vi "Copy Member Data from Target.vi"(7 "AppInst":refnum<vi>, 8 "error in (no error)":errorcluster, 11 "Target Method path":path) -> (0 "error out":errorcluster, 1 "Wiring Rules":T1(array[ring]), 2 "Controls[]":refnum<vi>[](array[refnum]), 3 "Target Method Ref":refnum<vi>)   [LabVIEW 2020, in "Message Maker.lvlib"]
uses:
  Message Maker.lvlib
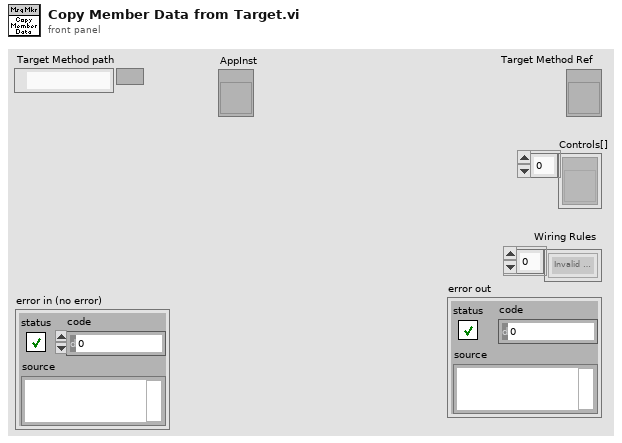
[diagram p1: front panel]
types:
  T1 = enum16{"Invalid Wire Rule", "Required", "Recommended", "Optional", "Dynamic Dispatch"}[]
  T2 = typedef "LVRectTypeDef.ctl" = cluster{"Left":i16, "Top":i16, "Right":i16, "Bottom":i16}
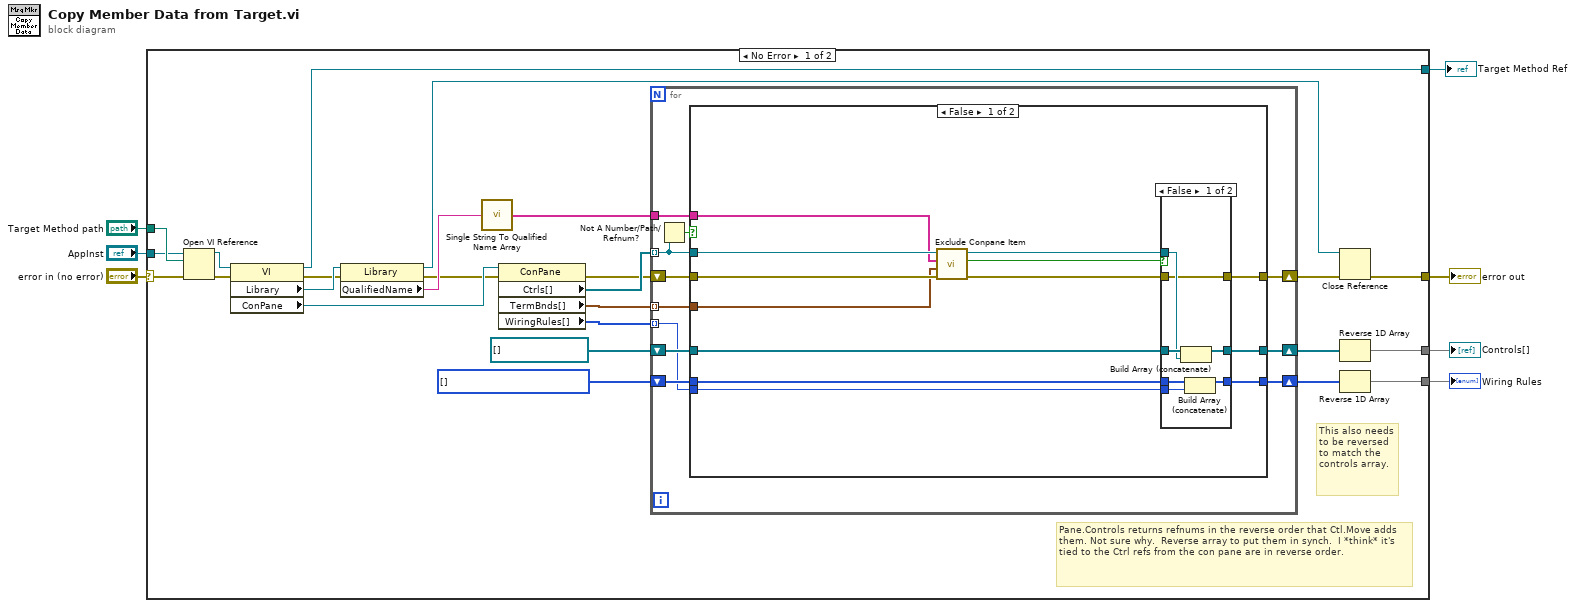
[diagram p0: block diagram]
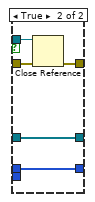
[diagram p2: hidden frame]
diagram:
  n1 = case shown="No Error" "error in (no error)" {
    selector: "error in (no error)" -> [w27 w72]
    tunnel: "Target Method path" -> [w28 _]
    tunnel: [w11 w72] -> w6
    tunnel: "AppInst" -> [w13 _]
    tunnel: [w8 _] -> w3
    tunnel: [w14 _] -> w2
    tunnel: [w12 _] -> w1
    frame No Error {
      w24 = T1 [] items=["Invalid Wire Rule", "Required", "Recommended", "Optional", "Dynamic Dispatch"] ("WiringRules[]")
      # "This also needs\nto be reversed to match the controls array."
      # "Pane.Controls returns refnums in the reverse order that Ctl.Move adds them. Not sure why.  Reverse array to put them in synch.  I *think* it's tied to the Ctrl refs from the con pane are in reverse order."
      n2 = Open VI Reference(application reference (local)=w13, vi path=w28, error in (no error)=w27) -> (vi reference=w29:refnum<vi>, error out=w30:errorcluster)  [unwired: 3 in]
      n3 = property class="VI"(reference=w29, error in=w30) -> (reference out=w12:refnum<vi>, error out=w31:errorcluster, "Library"=w32:refnum<vi>, "ConPane"=w22:refnum<vi>)
      n4 = property class="Library"(reference=w32, error in=w31) -> (reference out=w10:refnum<vi>, error out=w9:errorcluster, "QualifiedName"=w20:string)
      n5 = call <vilib>:"Single String To Qualified Name Array.vi"("Fully Qualified String"=w20) -> ("Fully Qualified Array"=w19:string[])
      n6 = property class="ConPane"(reference=w22, error in=w9) -> (error out=w18:errorcluster, "Ctrls[]"=w25:refnum<vi>[], "TermBnds[]"=w21:T2[], "WiringRules[]"=w23:T1)  [unwired: 1 out]
      n7 = for {
        tunnel: w25 -> [w38] mode=indexing
        tunnel: w19 -> [w43]
        shift-right: [w39] -> w17
        shift-left: w18 -> [w42]
        shift-right: [w40] -> w15
        shift-left: refnum<vi>[] [] ("Controls[]") -> [w41]
        shift-right: [w35] -> w16
        shift-left: w24 -> [w36]
        tunnel: w23 -> [w34] mode=indexing
        tunnel: w21 -> [w33] mode=indexing
        n8 = Not A Number/Path/Refnum?(number/path/refnum=w38) -> (NaN/Path/Refnum?=w37:bool)
        n9 = case shown="False" w37 {
          tunnel: w38 -> [w56 _]
          tunnel: w43 -> [w44 _]
          tunnel: w42 -> [w54 w71]
          tunnel: w41 -> [w52 w70]
          tunnel: [w51 w70] -> w40
          tunnel: [w50 w71] -> w39
          tunnel: w36 -> [w48 w69]
          tunnel: [w47 w69] -> w35
          tunnel: w34 -> [w46 _]
          tunnel: w33 -> [w45 _]
          frame False {
            n10 = call "Exclude Conpane Item.vi"("error in (no error)"=w54, "Rectangle"=w45, "Fully Qualified Array"=w44, "Control in"=w56) -> ("error out"=w53:errorcluster, "Exclude?"=w55:bool, "Control out"=w49:refnum<vi>)  [unwired: 5 in]
            n11 = case shown="False" w55 {
              tunnel: w49 -> [w61 w68]
              tunnel: w53 -> [w60 w67]
              tunnel: [w60 w66] -> w50
              tunnel: w52 -> [w63 w65]
              tunnel: [w62 w65] -> w51
              tunnel: w48 -> [w59 w64]
              tunnel: [w58 w64] -> w47
              tunnel: w46 -> [w57 _]
              frame False {
                n12 = Build Array (concatenate)(w63, w61) -> (w62:refnum<vi>[])
                n13 = Build Array (concatenate)(w59, w57) -> (w58:T1)
              }
              frame True {
                n14 = Close Reference(reference=w68, error in (no error)=w67) -> (error out=w66:errorcluster)
              }
            }
          }
          frame True {
          }
        }
      }
      n15 = Close Reference(reference=w10, error in (no error)=w17) -> (error out=w11:errorcluster)
      n16 = Reverse 1D Array(array=w15) -> (reversed array=w14:refnum<vi>[])
      n17 = Reverse 1D Array(array=w16) -> (reversed array=w8:T1)
    }
    frame Error {
    }
  }
  "error out" <- w6
  "Wiring Rules" <- w3
  "Controls[]" <- w2
  "Target Method Ref" <- w1
